vi "Secondary Loop.vi"(0 "Numeric 2":dbl, 1 "Numeric 3":dbl, 5 "Numeric":dbl, 7 "Sec Cold Temp (K)":dbl, 9 "Sec Mass Flow (kg/s) in":dbl, 12 "Sec Hot Temp (K) in":dbl) -> (3 "Secondary Cold Temperature (K)":dbl, 4 "Temperature (C) 2":dbl, 6 "Sec Mass Flow (kg/s) out":dbl, 8 "FLiNaK Ave Viscosity (Pa-s)":dbl, 10 "Sec Hot Temp (K) out":dbl, 13 "Secondary Average Temperature (C)":dbl, 14 "Temperature (C)":dbl)   [LabVIEW 2019]
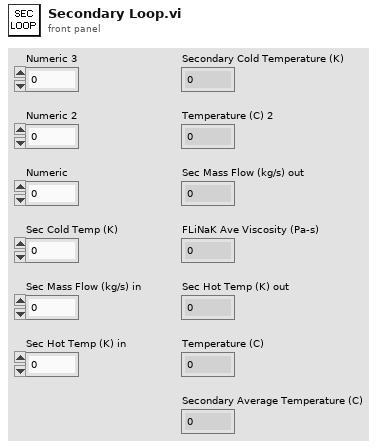
[diagram p1: front panel]
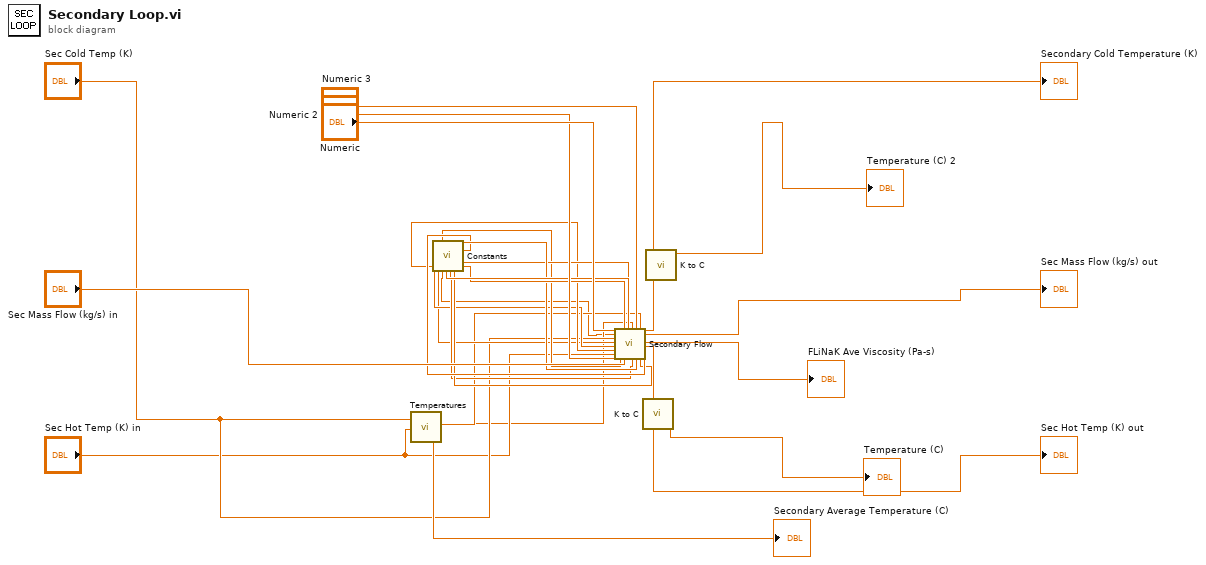
[diagram p0: block diagram]
diagram:
  n1 = call "Temperatures.vi"("Sec Cold Temp"="Sec Cold Temp (K)", "Sec Hot Temp"="Sec Hot Temp (K) in") -> ("Secondary Average Temperature (C)"=→"Secondary Average Temperature (C)":dbl, "Secondary Delta T (K)"=w2:dbl, "Secondary Average Temperature (K)"=w3:dbl)  [unwired: 7 in, 8 out]
  n2 = call "Constants.vi"() -> ("MHX Tube Pitch (m)"=w8:dbl, "Sec Loop Width (m)"=w7:dbl, "MHX Tube Diameter (m)"=w6:dbl, "Pipe Diameter (m)"=w9:dbl, "Dctl (m)"=w1:dbl, "Sec Loop Height (m)"=w16:dbl, "MHX Length (m)"=w11:dbl, "Number of MHX Baffles"=w12:dbl, "NDHX Tube Diameter (m)"=w14:dbl, "NDHX Tube Length (m)"=w13:dbl, "Pipe X-SectionArea (m^2)"=w10:dbl, "NDHX Number of Tubes"=w15:dbl)  [unwired: 5 in, 11 out]
  n3 = call "Secondary Flow.vi"("NDHX Heat Transfer (W)"="Numeric", "Dctl (m)"=w1, "Sec Cold Temp (K)"="Sec Cold Temp (K)", "MHX Tube Diameter (m)"=w6, "Sec Loop Width (m)"=w7, "MHX Tube Pitch (m)"=w8, "Sec Hot Temp (K)"="Sec Hot Temp (K) in", "MHX Heat Transfer (W)"="Numeric 2", "Pipe Diameter (m)"=w9, "NDHX Number of Tubes"=w15, "Sec Mass Flow (kg/s)"="Sec Mass Flow (kg/s) in", "Sec Loop Height (m)"=w16, "Pipe XArea (m^2)"=w10, "Sec Delta T (K)"=w2, "MHX Length (m)"=w11, "Time"="Numeric 3", "NDHX Tube Diameter (m)"=w14, "Sec Ave Temp (K)"=w3, "Number of MHX Baffles"=w12, "NDHX Tube Length (m)"=w13) -> ("Secondary Cold Temperature (K)"=w21:dbl, "Sec Mass Flow (kg/s)"=→"Sec Mass Flow (kg/s) out":dbl, "FLiNaK Ave Viscosity (Pa-s)"=→"FLiNaK Ave Viscosity (Pa-s)":dbl, "Sec Hot Temp (K)"=w22:dbl)  [unwired: 3 in, 1 out]
  "Sec Hot Temp (K) out" <- w22
  "Secondary Cold Temperature (K)" <- w21
  n4 = call "K to C.vi"("Temperature (K)"=w22) -> ("Temperature (C)"=→"Temperature (C)":dbl)  [unwired: 10 in]
  n5 = call "K to C.vi"("Temperature (K)"=w21) -> ("Temperature (C)"=→"Temperature (C) 2":dbl)  [unwired: 10 in]
